vi "Configurable PWM Tester - AO.vi"() -> ()   [LabVIEW 2021]
uses:
  <vilib>/Utility/error.llb/DialogType.ctl
  <vilib>/DAQmx/write.llb/DAQmx Write (Counter Frequency 1Chan 1Samp).vi
  <vilib>/DAQmx/configure/timing.llb/DAQmx Timing (Implicit).vi
  <vilib>/DAQmx/miscellaneous.llb/DAQmx Fill In Error Info.vi
  <vilib>/DAQmx/create/channels.llb/DAQmx Create Channel (CO-Pulse Generation-Frequency).vi
  <resource>/objmgr/daqmx.rc
panel:
  in  "duty cycle":dbl=0.1 min=0.05 max=0.1 format="%_6g"
  in  "stop":bool
  in  "Output Terminal":tag="/Dev1/PFI12"
  in  "Counter":tag="Dev1/ctr0"
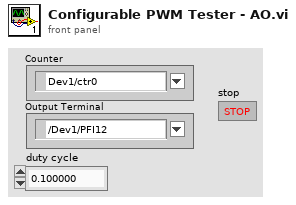
[diagram p1: front panel]
types:
  T1 = typedef "DialogType.ctl" = u16
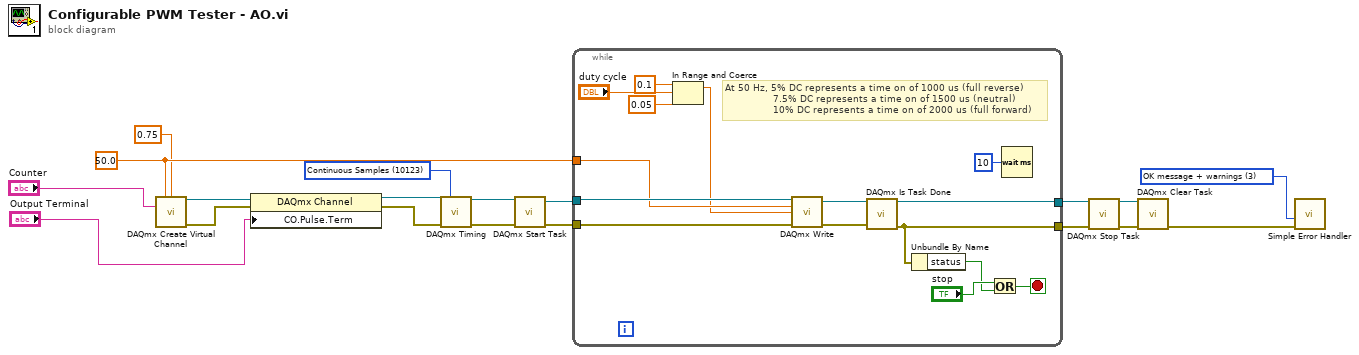
[diagram p0: block diagram]
diagram:
  w1 = 10123 items=["Finite Samples"=10178, "Continuous Samples"=10123, "Hardware Timed Single Point"=12522] ("sample mode")
  w8 = 50.0 ("Frequency")
  w16 = T1 3 items=["no dialog", "OK message", "continue or stop message", "OK message + warnings", "continue/stop + warnings"] ("type of dialog (OK msg:1)")
  n1 = call-poly <vilib>:"DAQmx Create Virtual Channel.vi"("frequency"=w8, "duty cycle"=0.75, "counter"="Counter") -> ("task out"=w6:refnum<k21>, "error out"=w5:errorcluster)  [unwired: 11 in]
  n2 = property class="DAQmx Channel"(reference=w6, error in=w5, "CO.Pulse.Term"="Output Terminal") -> (reference out=w4:refnum<k21>, error out=w3:errorcluster)
  n3 = call-poly <vilib>:"DAQmx Timing.vi"("task/channels in"=w4, "sample mode"=w1, "error in"=w3) -> ("task out"=w11:refnum<k21>, "error out"=w10:errorcluster)  [unwired: 11 in]
  n4 = call <vilib>:"DAQmx Start Task.vi"("task/channels in"=w11, "error in"=w10) -> ("task out"=w14:refnum<k21>, "error out"=w13:errorcluster)  [unwired: 12 in]
  n5 = while {
    tunnel: w13 -> [w28]
    tunnel: [w31] -> w15
    tunnel: w14 -> [w27]
    tunnel: [w30] -> w12
    tunnel: w8 -> [w26]
    stop <- w33 stop-if-true
    # "At 50 Hz, 5% DC represents a time on of 1000 us (full reverse)\n                7.5% DC represents a time on of 1500 us (neutral)\n                10% DC represents a time on of 2000 us (full forward)"
    n6 = In Range and Coerce(upper limit=0.1, x="duty cycle", lower limit=0.05) -> (coerced(x)=w20:dbl)  [unwired: 1 out]
    n7 = call-poly <vilib>:"DAQmx Write.vi"("task/channels in"=w27, "frequency"=w26, "duty cycle"=w20, "error in"=w28) -> ("task out"=w24:refnum<k21>, "error out"=w25:errorcluster)  [unwired: 9 in, 1 out]
    n8 = call <vilib>:"DAQmx Is Task Done.vi"("task/channels in"=w24, "error in"=w25) -> ("task out"=w31:refnum<k21>, "error out"=w30:errorcluster)  [unwired: 11 in, 1 out]
    n9 = Unbundle By Name(w30) -> ("status"=w32:bool)
    n10 = Or(x="stop", y=w32) -> (x .or. y?=w33:bool)
    n11 = Wait (ms)(milliseconds to wait=u32 10) -> ()  [unwired: 1 out]
  }
  n12 = call <vilib>:"DAQmx Stop Task.vi"("task/channels in"=w15, "error in"=w12) -> ("task out"=w18:refnum<k21>, "error out"=w17:errorcluster)  [unwired: 12 in]
  n13 = call <vilib>:"DAQmx Clear Task.vi"("task in"=w18, "error in"=w17) -> ("error out"=w19:errorcluster)  [unwired: 13 in]
  n14 = call <vilib>:"Simple Error Handler.vi"("type of dialog (OK msg:1)"=w16, "error in (no error)"=w19) -> ()  [unwired: 3 in, 5 out]
